vi "Process.vi"(8 "error in":errorcluster, 11 "Plugin in":refnum<class "Historical Table.lvclass">) -> (0 "error out":errorcluster, 3 "Plugin out":refnum<class "Historical Table.lvclass">)   [LabVIEW 2024, in "Historical Table.lvlib" / "Historical Table.lvclass"]
uses:
  Historical Table.lvclass
  <vilib>/FlexLogger/SDK/PluginSDK.lvlibp/PEFClasses/SDK/Plugin/Plugin.lvclass
  C:/Program Files/National Instruments/LabVIEW 2024/vi.lib/FlexLogger/SDK/PluginSDK.lvlibp/PEFClasses/SDK/Plugin/Plugin.lvclass
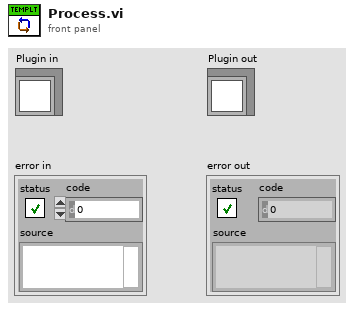
[diagram p1: front panel]
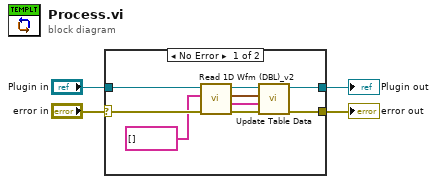
[diagram p0: block diagram]
diagram:
  n1 = case shown="No Error" "error in" {
    selector: "error in" -> [w13 w14]
    tunnel: [w6 w15] -> w1
    tunnel: "Plugin in" -> [w7 w15]
    tunnel: [w5 w14] -> w2
    frame No Error {
      n2 = call <vilib>:"Read 1D Wfm (DBL)_v2.vi"("error in (no error)"=w13, "Unique Identifers (empty = all)"=string[] [] ("Unique Channel Identifers (empty = all)"), "Plugin in"=w7) -> ("error out"=w8:errorcluster, "Stream Names"=w9:string[], "Data"=w10:waveform(dbl)[], "Plugin out"=w11:refnum<class "Historical Table.lvclass">)  [unwired: 5 in]
      n3 = call "Update Table Data.vi"("error in (no error)"=w8, "Stream Names"=w9, "Data"=w10, "Plugin in"=w11) -> ("error out"=w5:errorcluster, "Plugin out"=w6:refnum<class "Historical Table.lvclass">)  [unwired: 6 in]
    }
    frame Error {
    }
  }
  "error out" <- w2
  "Plugin out" <- w1
